vi "Chart.vi"() -> ()   [LabVIEW 2014]
panel:
  out "Chart":dbl(graph)
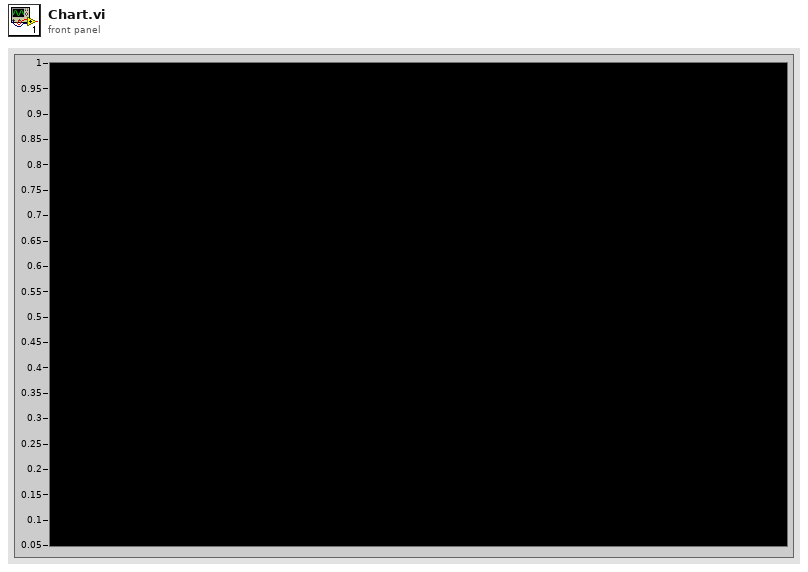
[diagram p1: front panel]
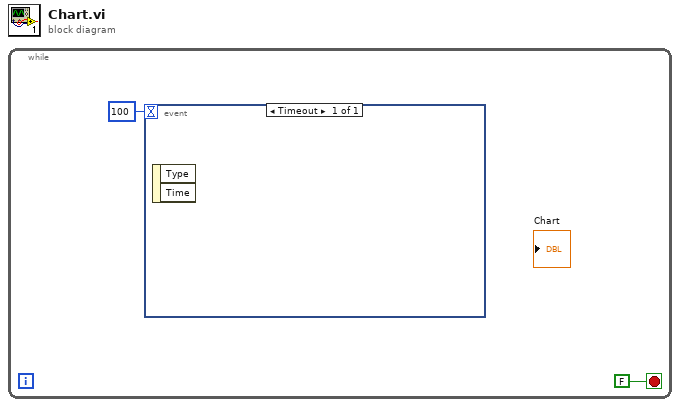
[diagram p0: block diagram]
diagram:
  n1 = while {
    stop <- FALSE stop-if-true
    n2 = event shown="[0] Timeout" {
      selector: _ -> [_]
      dyn-events: _ -> [_]
      timeout: 100 -> [_]
      event Timeout {
        n3 = event-data() -> ()  [unwired: 1 in, 2 out]
      }
    }
  }
